vi "Query Generator ARB File Option.vi"(8 "error in (no error)":errorcluster, 10 "Instance (1)":i32=1, 11 "VISA resource name":refnum<visa-resource-name>) -> (0 "error out":errorcluster, 2 "File Option":string, 3 "VISA resource name out":refnum<visa-resource-name>)   [LabVIEW 2020, in "Rohde&Schwarz CMXP GPRF.lvlib"]
doc: "Queries the R&S CMW-KV and R&S CMW-KW-options that are required to process the loaded ARB file with the arbitrary RF generator.\n\nAttribute:\nRSCMXPGPRF_ATTR_ARB_FILE_OPTION\n\nRemote-control command:\nSOURce:GPRF:GEN<i>:ARB:FILE:OPTion?"
uses:
  <instrlib>/Rohde&Schwarz CMXP GPRF/Rohde&Schwarz CMXP GPRF.lvlib
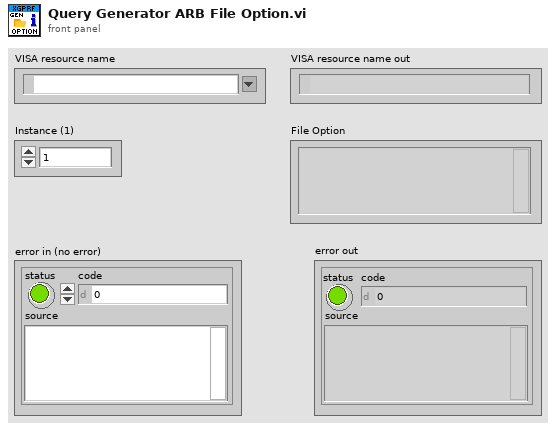
[diagram p1: front panel]
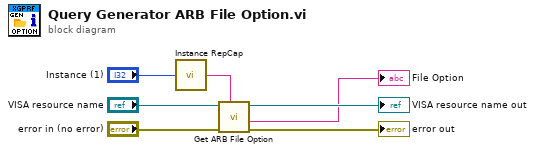
[diagram p0: block diagram]
diagram:
  n1 = call <instrlib>:"Instance RepCap.vi"("Instance in"="Instance (1)") -> ("Instance out"=w7:string)
  n2 = call "Get ARB File Option"("Repeated Capabilities"=w7, "error in (no error)"="error in (no error)", "instrument handle"="VISA resource name") -> ("error out"=→"error out":errorcluster, "ARB File Option"=→"File Option":string, "instrument handle out"=→"VISA resource name out":refnum<visa-resource-name>)  [unwired: 6 in]
